vi "init control_string.vi"(10 "Str Refnum":refnum<vi>) -> (2 "Control out":refnum<class "Control.lvclass">)   [LabVIEW 2010, in "Control.lvclass"]
uses:
  Control.lvclass
  String Control/String Control.lvclass
  Control.lvclass/Control.ctl
panel:
  in  "Control in":refnum<class "Control.lvclass">
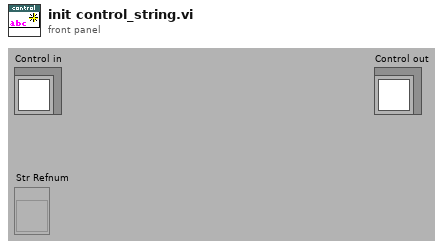
[diagram p1: front panel]
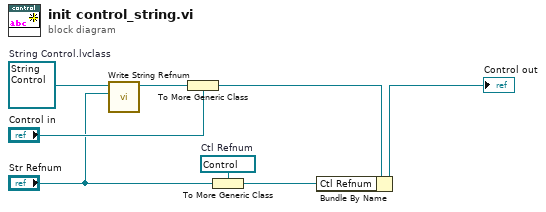
[diagram p0: block diagram]
diagram:
  w5 = refnum<vi> refnum  # Ctl Refnum
  w3 = refnum<class "String Control.lvclass"> refnum  # String Control.lvclass
  n1 = call "Write String Refnum.vi"("String Refnum"="Str Refnum", "String Control in"=w3) -> ("String Control out"=w2:refnum<class "String Control.lvclass">)  [unwired: 8 in, 1 out]
  n2 = To More Generic Class(target class="Control in", reference=w2) -> (generic class reference=w4:refnum<class "Control.lvclass">)
  n3 = To More Generic Class(target class=w5, reference="Str Refnum") -> (generic class reference=w6:refnum<vi>)
  n4 = Bundle By Name(cluster=w4, "Ctl Refnum"=w6) -> (→"Control out":refnum<class "Control.lvclass">)
